vi "GetStatus.vi"() -> ()   [LabVIEW 2018]
doc: "Use this template to build a user interface event handler design pattern. Use this pattern for dialog boxes and other user interfaces. You also can create and execute user-defined events that the VI can handle the same way as user interface events."
panel:
  out "status":bool
  out "Numeric":i32
  in  "Button 1":bool
  in  "stop":bool
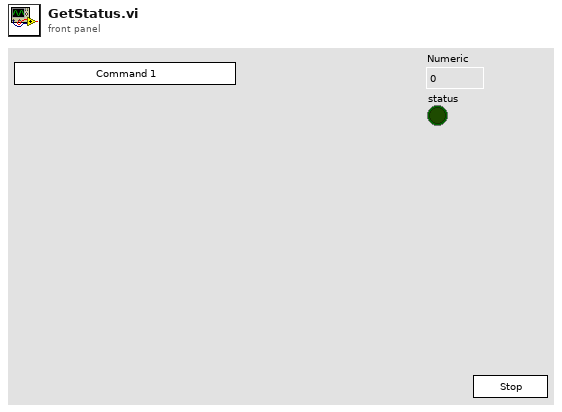
[diagram p1: front panel]
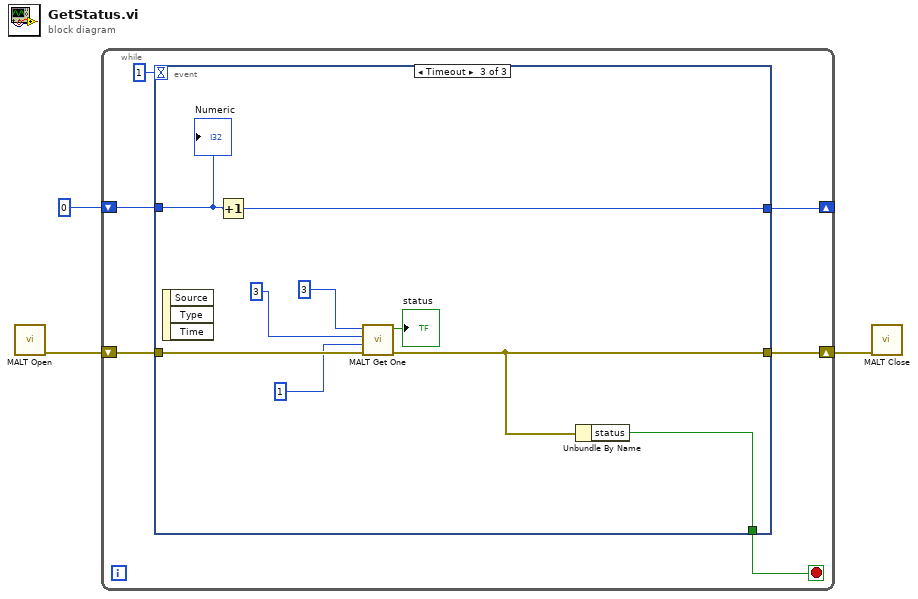
[diagram p0: block diagram]
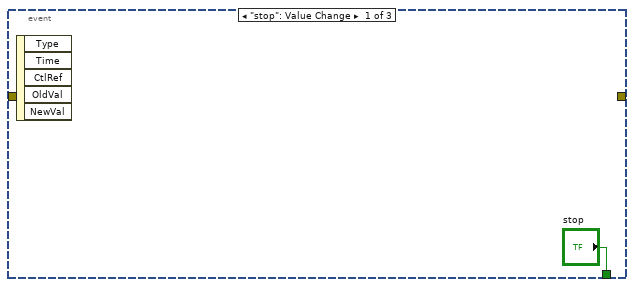
[diagram p2: hidden frame]
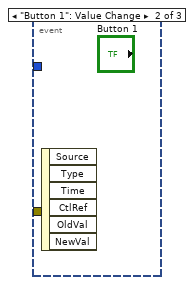
[diagram p3: hidden frame]
diagram:
  n1 = call "MALT Open.vi"() -> ("error out"=w3:errorcluster)  [unwired: 11 in]
  n2 = while {
    shift-right: [w6] -> w2
    shift-left: w3 -> [w7]
    shift-right: [w4] -> _
    shift-left: 0 -> [w5]
    stop <- w9 stop-if-true
    n3 = event shown="[2] Timeout" {
      selector: _ -> [_ _ _]
      dyn-events: _ -> [_ _ _]
      timeout: 1 -> [_ _ _]
      tunnel: ["stop" _ w17] -> w9
      tunnel: w7 -> [_ _ w19]
      tunnel: [_ _ w18] -> w6
      tunnel: w5 -> [_ _ w13]
      tunnel: [_ _ w12] -> w4
      event "stop": Value Change {
        n4 = event-data() -> ()  [unwired: 1 in, 5 out]
      }
      event "Button 1": Value Change {
        n5 = event-data() -> ()  [unwired: 1 in, 6 out]
      }
      event Timeout {
        n6 = event-data() -> ()  [unwired: 1 in, 3 out]
        n7 = Increment(x=w13) -> (x+1=w12:i32)
        n8 = call "MALT Get One.vi"("error in"=w19, "port"=1 ("Port"), "address"=3 ("Address"), "cardType"=3 ("CardType")) -> ("error out"=w18:errorcluster, "status"=→"status":bool)  [unwired: 6 in]
        n9 = Unbundle By Name(w18) -> ("status"=w17:bool)
        "Numeric" <- w13
      }
    }
  }
  n10 = call "MALT Close.vi"("error in"=w2) -> ()  [unwired: 10 in, 1 out]
